vi "Big_LED_control.vi"() -> ()   [LabVIEW 2018]
uses:
  <instrlib>/niDCPower/nidcpower.llb/niDCPower Source Mode.ctl
  <instrlib>/niDCPower/nidcpower.llb/niDCPower Output Function.ctl
  AT lib/AmateurStepperMotor.dll
  <instrlib>/niDMM/nidmm.llb/niDMM Function.ctl
  <instrlib>/niDMM/nidmm.llb/niDMM Resolution in Digits.ctl
  <vilib>/Instr/_visa.llb/VISA Configure Serial Port (Instr).vi
  <instrlib>/niDMM/nidmm.llb/niDMM Configure Measurement Digits.vi
panel:
  in  "I - IV":bool
  in  "IV (gh)":bool
  in  "III (jk)":bool
  in  "II (Lm)":bool
  in  "I (np)":bool
  in  "Tab Control 2":enum32{"Шаговик и офир", "Служебная область"}(tab)
  in  "milliseconds to wait":u32=1000
  in  "Go To":dbl
  out "Ophir 1 Char":dbl(graph)=0.01
  in  "DecelerationTime, s":dbl=0.3
  in  "AccelerationTime, s":dbl=0.3
  in  "HoldOn":bool
  in  "Ophir 1 units":string(combo)="1000" caption="Units"
  out "Ophir 1 Over Range":bool caption="Over Range"
  out "Ophir 1 Optical Power":dbl=0.01 caption="Power" format="%#_4g"
  out "Ophir 1 MAX":dbl=0.01 caption="MAX" format="%#_5g"
  in  "Ophir 1 Clear":bool caption="Clear"
  in  "StepMultiplicationFactor":dbl=50.0
  in  "StepDivisor":i32(ring)=8 items=["D1"=1, "D2"=2, "D4"=4, "D8"=8, "D16"=16, "D32"=32]
  in  "Speed":dbl=250.0
  in  "Погнали!":bool
  in  "Стоп GoTo":bool
  out "Готово":bool
  out "Position":dbl=9.995
  in  "Ophir 1 Info":u16(ring)=1 caption="Info" items=["Device : JUNO; s/n:903793", "Head : PD300R-3W   ; s/n:779628"]
  in  "new pos":dbl
  in  "set pos":bool
  out "Device Response":string="*\n"
  in  "Ophir 1 usb channel":i16 caption="usb channel"
  out "Ophir 1 dup Visa Session":refnum<visa-resource-name>="USB0::0x0BD3::0x0777::NI-VISA-60003::RAW" caption="dup Visa Session"
  in  "Ophir 1 Baud Rate (3:9600)":i16(ring)=3 caption="Baud Rate (3:9600)" items=["300", "1200", "4800", "9600", "19200", "38400"]
  out "Ophir 1 Real Optical Power":dbl=1e-05 format="%.6e"
  in  "Ophir 1 GPIB Address (10)":string="10" caption="GPIB Address (10)"
  in  "Ophir 1 Port Number (default 2)":i16=1 caption="Port Number (default 2)" min=0 max=20
  in  "Ophir 1 Select Communication Protocol":u16(ring) caption="Select Communication Protocol" items=["USB", "RS232", "GPIB"]
  out "Ophir 1 error out":errorcluster caption="error out"
  in  "Ophir 1 error in (no error)":errorcluster caption="error in (no error)"
  in  "Ophir 1 Wait":u32=100 caption="Wait"
  out "IsOpen":bool=TRUE
  out "Ophir 1 Initialization":bool=TRUE caption="Initialization"
  in  "Tab Control":T1(tab)
  in  "POWER":bool
  in  "Стоп":bool
  in  "Resource Name":refnum<k15>="PXI1Slot2" caption="Источник питания"
  in  "Амперметр":refnum<k15>="PXI1Slot4" caption="NI DMM 1"
  in  "V_MB, V":dbl=6.0 caption="voltage level" min=0.0 max=6.0 format="%_6p"
  in  "curlim_V_MB, A":dbl=0.3 caption="current limit" format="%_6p"
  out "chart_0":dbl(graph)=-0.00013853853853977013 caption="Waveform Chart 5"
  in  "voltlim_I_LED, V":dbl=2.1 caption="current limit" min=0.01 format="%_6p"
  in  "I_LED, A":dbl=0.010000000000000004 caption="voltage level" format="%_6p"
  out "chart_1":dbl(graph)=-0.0002744397184121777 caption="Waveform Chart 5"
  out "Current Char":dbl(graph)=0.0055655837059021
  in  "Arduino":refnum<visa-resource-name>="COM16"
  in  "Сегменты":bool[](array[boolean])=[FALSE, FALSE, FALSE, FALSE, FALSE, FALSE, FALSE, FALSE, FALSE, FALSE, FALSE, FALSE, FALSE, FALSE, FALSE, FALSE, FALSE, FALSE]
  in  "Вольтметр":refnum<k15>="PXI1Slot5" caption="NI DMM 1"
  out "Voltage Char":dbl(graph)=0.2558511793613434
  in  "Port Name":string="COM8" caption="Порт шаговика"
  in  "wave_lenght":string="600"
  in  "Промер":bool caption="Промер сегмента"
  in  "NI DMM 1 Voltage Range 4":string(combo)="-1" caption="Range"
  in  "NI DMM 1 units 4":string(combo)="1" caption="Units"
  out "Voltage":dbl=0.2558511793613434 format="%_6g"
  in  "NI DMM 1 Current Range 3":string(combo)="1" caption="Range"
  in  "NI DMM 1 units 3":string(combo)="1000" caption="Units"
  out "Current":dbl=0.0055655837059021 format="%_6g"
  out "voltmes_V_MB, V":dbl=-0.00013853853853977013 caption="measurement" format="%_6g"
  out "curmes_V_MB, A":dbl=-0.0019423252169001965 caption="measurement" format="%_6g"
  out "curmes_I_LED, A":dbl=9.117163901385412e-07 caption="measurement" format="%_6g"
  out "voltmes_I_LED, V":dbl=-0.0002744397184121777 caption="measurement" format="%_6g"
  out "Разряд":dbl
  out "+/-":bool
  out "Power off":bool
  in  "Command":string="Cathode"
  in  "Записать":bool
  out "measure output \nfile refnum":refnum<file>
  out "Voltage, V":dbl=0.2558511793613434 caption="Measurement" format="%.5f"
  out "Current, A":dbl=5.5655837059021e-06 caption="Measurement" format="%.5f"
  out "Тип индикатора":string="Cathode"
  out "chart_2":dbl(graph)=0.0007584113885058215
  in  "V_RES, V":dbl caption="voltage level" format="%_6p"
  out "curmes_V_RES, A":dbl=9.838948216702391e-07 caption="measurement" format="%_6g"
  in  "curlim_V_RES, A":dbl=0.1 caption="current limit" min=0.01 format="%_6p"
  in  "measure path":path=path "C:/Users/user/Desktop/МСП/LabVIEW/LED_CONTROL_big_LED_ophir_24.12.24_1/Logs"
  out "Enum":enum16{"Exit", "4", "Промер", "2", "1"}(ring)
  out "№ об-ца":dbl
  out "Темп-ра":dbl
  out "Сегмент":string="n"
  out "voltmes_V_RES, V":dbl=0.0007584113885058215 caption="measurement" format="%_6g"
  in  "current level range":dbl=0.001 format="%#.6p"
  in  "1 - до 10 мА\n0 - от  30 мА":bool
  # "24.067"
  # "Шаговик"
  # "Офир"
  # "Шаговик"
  # "Офир"
  # "position - это значение абсолютное"
  # "j"
  # "c"
  # "d"
  # "e"
  # "g"
  # "h"
  # "a"
  # "b"
  # "f"
  # "k"
  # "L"
  # "m"
  # "n"
  # "p"
  # "dp"
  # "all"
  # "V_MB 5 В\nогрничение 300 м\n\nV_LED 2,1 В\nограничение 200 м"
  # "единицы мА\nrange 1 А"
  # "1. каждый сегмент включаем по отдельности, резистором постраиваем ток до 10 мА\n2. напряжение V_LED при этом не меняется\n3. в такоом положении промеряем сегменты по отдельности\n4. для промера всего индикатора сразу подстраиваем напряжение при неизменном положении резисторов\n5. ток всех индикаторов = ток одного сегмента (10 мА) * число сегментов (15)\n6. добиваемся этого увеличением V_LED"
  # "единицы В\nrange AUTO"
  # "регклировка суммарного тока через индикатор"
  # "24.063\n\n     I          U\n20 мА  1.3 В\n20 мА  1.4 В\n 7 мА   1.15 В"
  # "24.064\n\n     I          U\n10 мА  2 В\n10 мА  2.15 В\n 7 мА   1.9 В"
  # "автоматизировать подбор напряжения по известному максимальному напряжению и току. ОС по току сегмента"
  # "Р1:  +25°C\nР2:  - 60°C\nР3:  +85°C"
  # "регулировать ток в зависимости от температуры.\nс ростом температуры растет ток.\nпид-регулятор??"
  # "0. ввести номер образца\n1. включить нужный сегмент\n2. ввести его в поле справа\n3. вести температуру в поле слева\n4. нажать кнопку \"промер сегмента\""
  # "\"опрашивать кнопки не чаще, чем раз в секунду. сейчас кликать можно чаще, они загорятся, но ничего не произойдет\""
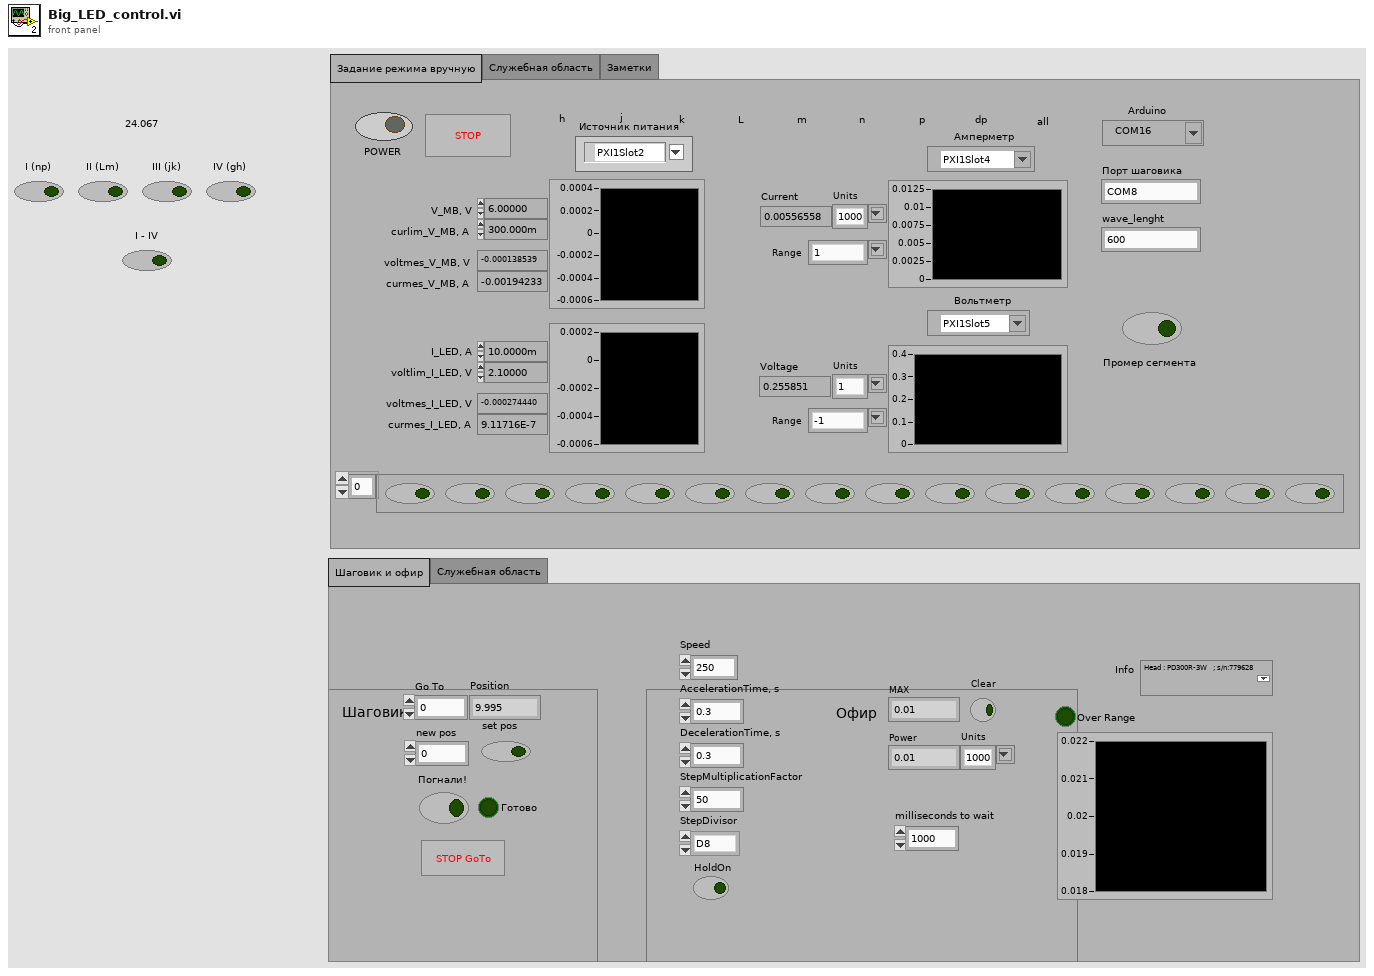
[diagram p1: front panel]
types:
  T1 = enum32{"Задание режима вручную", "Служебная область", "Заметки"}
  T2 = enum16{"open", "replace", "create", "open or create", "replace or create", "replace or create with confirmation"}
  T3 = typedef "niDCPower Output Function.ctl" = i32
  T4 = typedef "niDCPower Source Mode.ctl" = i32
  T5 = typedef "niDMM Function.ctl" = enum16{"DC Volts", "AC Volts", "DC Current", "AC Current", "2-wire Resistance", "4-wire Resistance", "Diode", "Frequency", "Period", "AC Volts DC Coupled", "Capacitance", "Inductance", "Temperature"}
  T6 = typedef "niDMM Resolution in Digits.ctl" = dbl
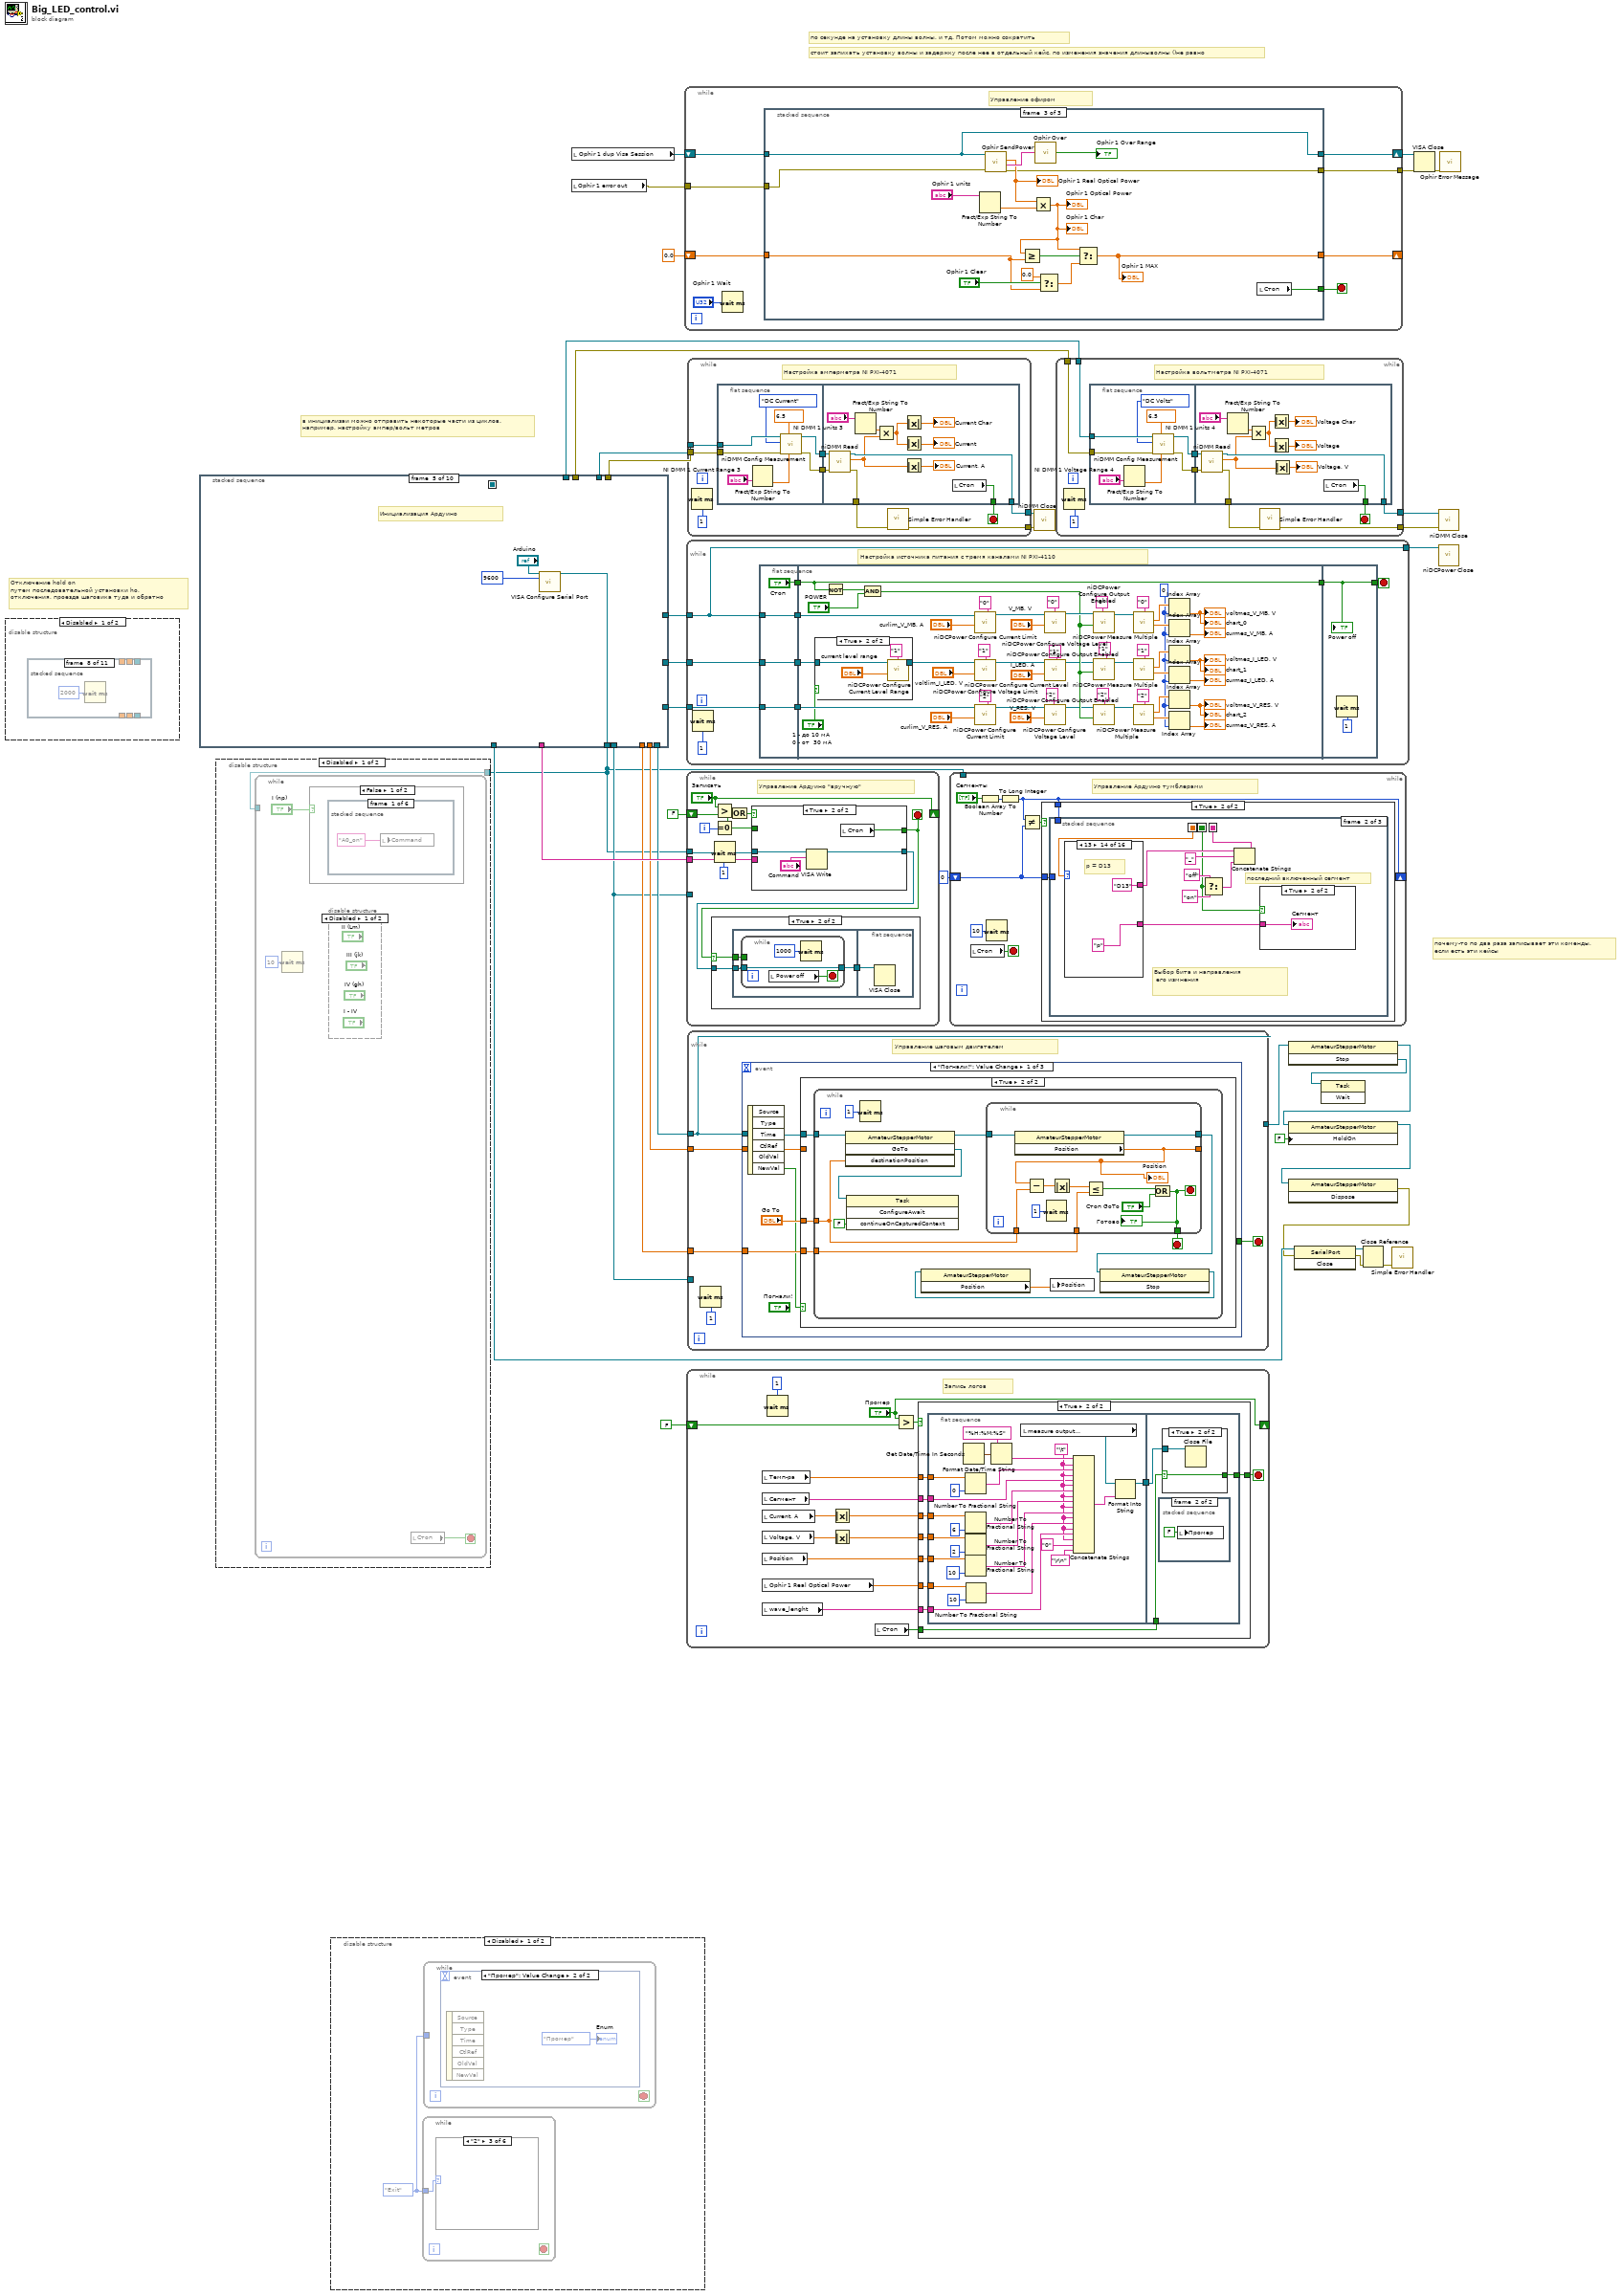
[diagram p0: block diagram]
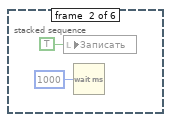
[diagram p3: hidden frame]
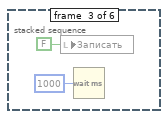
[diagram p4: hidden frame]
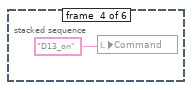
[diagram p5: hidden frame]
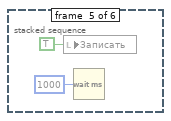
[diagram p6: hidden frame]
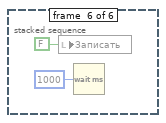
[diagram p7: hidden frame]
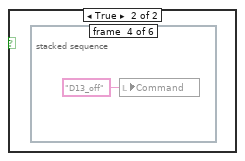
[diagram p8: hidden frame]
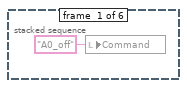
[diagram p9: hidden frame]
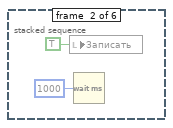
[diagram p10: hidden frame]
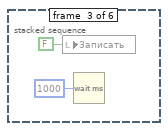
[diagram p11: hidden frame]
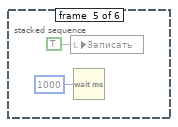
[diagram p12: hidden frame]
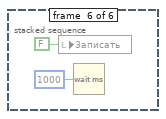
[diagram p13: hidden frame]
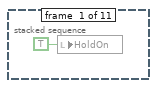
[diagram p15: hidden frame]
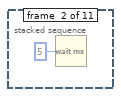
[diagram p16: hidden frame]
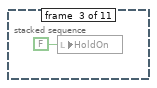
[diagram p17: hidden frame]
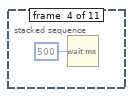
[diagram p18: hidden frame]
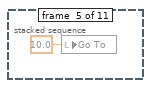
[diagram p19: hidden frame]
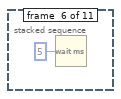
[diagram p20: hidden frame]
diagram:
  # "почему-то по два раза записывает эти коменды,\nесли есть эти кейсы"
  # "Отключение hold on\nпутем последовательной установки ho, \nотключения, проезда шаговика туда и обратно"
  # "в инициализаи можно отправить некоторые части из циклов.\nнапример, настройку ампер/вольт метров"
  # "стоит запихать установку волны и задержку после нее в отдельный кейс, по изменения значения длиныволны ()не равно"
  # "по секунде на установку длины волны, и тд. Потом можно сократить"
  n1 = disable-structure shown="Disabled" {
    frame Disabled {
      n2 = stacked-sequence {
        tunnel: _ -> [_ _ _ _ _ _ _ _ _ _ w50]
        tunnel: [_ _ _ _ _ _ _ _ _ _ w50] -> _
        tunnel: _ -> [_ _ _ _ _ _ _ _ _ _ w49]
        tunnel: [_ _ _ _ _ _ _ _ _ _ w49] -> _
        tunnel: [_ _ _ _ _ _ _ _ _ _ w48] -> _
        tunnel: _ -> [_ _ _ _ _ _ _ _ _ _ w48]
        frame #0 {
          n3 = local write "HoldOn"(TRUE ("HoldOn")) -> ()
        }
        frame #1 {
          n4 = Wait (ms)(milliseconds to wait=u32 5) -> ()  [unwired: 1 out]
        }
        frame #2 {
          n5 = local write "HoldOn"(FALSE ("HoldOn")) -> ()
        }
        frame #3 {
          n6 = Wait (ms)(milliseconds to wait=u32 500) -> ()  [unwired: 1 out]
        }
        frame #4 {
          n7 = local write "Go To"(10.0 ("Go To")) -> ()
        }
        frame #5 {
          n8 = Wait (ms)(milliseconds to wait=u32 5) -> ()  [unwired: 1 out]
        }
        frame #6 {
          n9 = local write "Погнали!"(TRUE ("Погнали!")) -> ()
        }
        frame #7 {
          n10 = Wait (ms)(milliseconds to wait=u32 2000) -> ()  [unwired: 1 out]
        }
        frame #8 {
          n11 = local write "Go To"(0.0 ("Go To")) -> ()
        }
        frame #9 {
          n12 = Wait (ms)(milliseconds to wait=u32 5) -> ()  [unwired: 1 out]
        }
        frame #10 {
          n13 = local write "Погнали!"(TRUE ("Погнали!")) -> ()
        }
      }
    }
    frame Enabled {
    }
  }
  n14 = stacked-sequence {
    seq-local: [_ _ _ _ _ _ w121 _ _ _] -> [_ _ _ _ _ _ _ w130 _ _]
    tunnel: [_ _ _ w68 _ _ _ _ _ _] -> w26
    tunnel: [_ w62 _ _ _ _ _ _ _ _] -> w37
    tunnel: [_ w61 _ _ _ _ _ _ _ _] -> w36
    tunnel: [_ _ _ _ w88 _ _ _ _ _] -> w1
    tunnel: [_ _ _ _ _ _ _ _ w136 _] -> w33
    tunnel: [_ _ w65 _ _ _ _ _ _ _] -> w32
    tunnel: [_ _ w64 _ _ _ _ _ _ _] -> w31
    tunnel: [_ _ _ _ _ _ _ w133 _ _] -> w3
    tunnel: [_ _ _ _ _ _ _ w131 _ _] -> w4
    tunnel: [_ _ _ _ _ _ _ w132 _ _] -> w5
    tunnel: [_ _ _ _ _ _ w111 _ _ _] -> w20
    tunnel: [_ _ _ w67 _ _ _ _ _ _] -> w8
    tunnel: [_ _ _ w66 _ _ _ _ _ _] -> w6
    tunnel: [_ _ _ _ _ _ _ _ _ w137] -> w2
    frame #0 {
      w52 = 0.0 ("currentmes_2")
      w53 = FALSE ("Стоп")
      # "ch 1"
      # "Обнуление переменных"
      n15 = local write "POWER"(w53) -> ()
      n16 = local write "Стоп"(w53) -> ()
      n17 = local write "+/-"(w53) -> ()
      n18 = local write "Погнали!"(w53) -> ()
      n19 = local write "Готово"(w53) -> ()
      n20 = local write "Стоп GoTo"(w53) -> ()
      n21 = local write "Промер"(w53) -> ()
      n22 = local write "curmes_V_MB, A"(w52) -> ()
      n23 = local write "voltmes_I_LED, V"(w52) -> ()
      n24 = local write "curmes_V_RES, A"(w52) -> ()
      n25 = local write "Current"(w52) -> ()
      n26 = local write "Разряд"(w52) -> ()
      n27 = local write "Go To"(w52) -> ()
      n28 = local write "Темп-ра"(w52) -> ()
      n29 = local write "№ об-ца"(w52) -> ()
      n30 = local write "Speed"(250.0 ("Speed")) -> ()
      n31 = local write "StepMultiplicationFactor"(50.0 ("StepMultiplicationFactor")) -> ()
      n32 = local write "AccelerationTime, s"(0.3 ("AccelerationTime, s")) -> ()
      n33 = local write "DecelerationTime, s"(0.3 ("DecelerationTime, s")) -> ()
      n34 = local write "current level range"(0.001 ("current level range")) -> ()
      n35 = local write "Сегменты"(bool[] [FALSE, FALSE, FALSE, FALSE, FALSE, FALSE, FALSE, FALSE, FALSE, FALSE, FALSE, FALSE, FALSE, FALSE, FALSE, FALSE, FALSE, FALSE] ("Сегменты")) -> ()
    }
    frame #1 {
      # "Инициализация амперметра"
      n36 = call <instrlib>:"niDMM Initialize.vi"("Instrument Descriptor"="Амперметр") -> ("error out"=w62:errorcluster, "instrument handle out"=w61:refnum<k15>)  [unwired: 9 in]
    }
    frame #2 {
      # "Инициализация вольтметра"
      n37 = call <instrlib>:"niDMM Initialize.vi"("Instrument Descriptor"="Вольтметр") -> ("error out"=w64:errorcluster, "instrument handle out"=w65:refnum<k15>)  [unwired: 9 in]
    }
    frame #3 {
      w73 = T3 1006 items=["DC Voltage"=1006, "DC Current"=1007, "Pulse Voltage"=1049, "Pulse Current"=1050] ("output function")
      w77 = T3 1007 items=["DC Voltage"=1006, "DC Current"=1007, "Pulse Voltage"=1049, "Pulse Current"=1050] ("output function")
      w78 = T3 1006 items=["DC Voltage"=1006, "DC Current"=1007, "Pulse Voltage"=1049, "Pulse Current"=1050] ("output function")
      w81 = T4 1020 items=["Single Point"=1020, "Sequence"=1021] ("source mode")
      # "Инициализация источника питания"
      n38 = call <instrlib>:"niDCPower Initialize.vi"("resource name"="Resource Name") -> ("instrument handle out"=w82:refnum<k15>)  [unwired: 3 in, 7 out]
      n39 = call <instrlib>:"niDCPower Configure Source Mode.vi"("source mode"=w81, "instrument handle"=w82) -> ("instrument handle out"=w72:refnum<k15>)  [unwired: 1 in, 8 out]
      n40 = call <instrlib>:"niDCPower Configure Output Function.vi"("output function"=w77, "channel name"="1", "instrument handle"=w72) -> ("instrument handle out"=w79:refnum<k15>)  [unwired: 7 in, 1 out]
      n41 = call <instrlib>:"niDCPower Configure Output Function.vi"("output function"=w73, "channel name"="2", "instrument handle"=w72) -> ("instrument handle out"=w74:refnum<k15>)  [unwired: 7 in, 1 out]
      n42 = call <instrlib>:"niDCPower Configure Output Function.vi"("output function"=w78, "channel name"="0", "instrument handle"=w72) -> ("instrument handle out"=w80:refnum<k15>)  [unwired: 7 in, 1 out]
      n43 = call <instrlib>:"niDCPower Configure Voltage Level.vi"("voltage level"=0.0, "channel name"="2", "instrument handle"=w74) -> ("instrument handle out"=w66:refnum<k15>)  [unwired: 7 in, 1 out]
      n44 = call <instrlib>:"niDCPower Configure Voltage Level.vi"("voltage level"=0.0, "channel name"="0", "instrument handle"=w80) -> ("instrument handle out"=w68:refnum<k15>)  [unwired: 7 in, 1 out]
      n45 = call <instrlib>:"niDCPower Configure Current Level.vi"("current level"=0.01, "channel name"="1", "instrument handle"=w79) -> ("instrument handle out"=w67:refnum<k15>)  [unwired: 7 in, 1 out]
    }
    frame #4 {
      # "Инициализация Ардуино"
      n46 = call-poly "VISA Configure Serial Port"("VISA resource name"="Arduino", "baud rate (9600)"=u32 9600) -> ("VISA resource name out"=w88:refnum<visa-resource-name>)  [unwired: 12 in, 1 out]
    }
    frame #5 {
      # "Инициализация офира"
      n47 = call "Ophir InitCom.vi"("GPIB Address (default 10)"="Ophir 1 GPIB Address (10)", "Communication (default USB 0)"="Ophir 1 Select Communication Protocol", "USB Channel number (default 0)"="Ophir 1 usb channel", "Port Number (default 2)"="Ophir 1 Port Number (default 2)", "error in (no error)"="Ophir 1 error in (no error)", "Baud Rate (3:9600)"="Ophir 1 Baud Rate (3:9600)") -> ("dup Visa Session"=w97:refnum<visa-resource-name>, "error out"=w96:errorcluster)  [unwired: 1 out]
      n48 = call "Ophir InstrInfo.vi"("Visa Session"=w97, "error in (no error)"=w96) -> ("dup Visa Session"=w109:refnum<visa-resource-name>, "Instrument Info"=w91:string, "error out"=w107:errorcluster)
      n49 = call "Ophir HeadInfo.vi"("Visa Session"=w109, "error in (no error)"=w107) -> ("error out"=w106:errorcluster, "dup Visa Session"=w108:refnum<visa-resource-name>, "Head Info"=w105:string)  [unwired: 6 out]
      n50 = call "Ophir InfoStrings.vi"("error in (no error)"=w106, "Head Info"=w105, "Instrument Info"=w91) -> ("error out"=w104:errorcluster, "Strings Array"=w103:string[])
      n51 = property on="Ophir 1 Info" class="Ring (strict)"("Strings []"=w103) -> ()  [unwired: 2 in, 2 out]
      n52 = call "Ophir ConfigDevice.vi"("Visa Session"=w108, "Measure Choice (0:Power)"=u16 0, "error in (no error)"=w104) -> ("dup Visa Session"=→"Ophir 1 dup Visa Session":refnum<visa-resource-name>, "OK ?"=→"Ophir 1 Initialization":bool, "error out"=→"Ophir 1 error out":errorcluster)  [unwired: 1 out]
    }
    frame #6 {
      w115 = 100 ("WriteTimeout")
      w120 = 1 items=["None", "One", "Two", "OnePointFive"] ("stopBits")
      w117 = 0 items=["None", "Odd", "Even", "Mark", "Space"] ("parity")
      # "убрали открытие порта. шаговик его и так сам откроет"
      # "Инициализация шаговика ч.1"
      n53 = constructor class="SerialPort"("portName"="Port Name", "baudRate"=57600, "parity"=w117, "dataBits"=8, "stopBits"=w120) -> (reference out=w114:refnum<k24>, error out=w113:errorcluster)  [unwired: 3 in, 6 out]
      n54 = property class="SerialPort"(reference=w114, error in=w113, "WriteTimeout"=w115, "ReadTimeout"=w115) -> (reference out=w111:refnum<k24>)  [unwired: 1 out]
      n55 = constructor class="AmateurStepperMotor"("serialPort"=w111) -> (reference out=w121:refnum<k24>, error out=w112:errorcluster)  [unwired: 3 in, 2 out]
      n56 = flat-sequence {
        tunnel: w112 -> [_]
        tunnel: w111 -> [w123]
        frame #0 {
          n57 = property class="SerialPort"(reference=w123) -> ("IsOpen"=→"IsOpen":bool)  [unwired: 1 in, 2 out]
        }
      }
    }
    frame #7 {
      # "стоит допустить изменение\nтих параметров в цикле, а не только \nпри инициализации"
      # "это те самые 50 шагов за мм"
      # "Инициализация шаговика ч.2"
      n58 = property class="AmateurStepperMotor"(reference=w130, "Speed"="Speed", "StepDivisor"="StepDivisor", "StepMultiplicationFactor"="StepMultiplicationFactor", "AccelerationTime"="AccelerationTime, s", "DecelerationTime"="DecelerationTime, s", "HoldOn"="HoldOn") -> (reference out=w133:refnum<k24>, "Position"=w131:dbl, "PositioningPrecision"=w132:dbl)  [unwired: 1 in, 1 out]
    }
    frame #8 {
      # "Begin VI: ОК или ОА?"
      n59 = call "Begin.vi"() -> ("Темп-ра"=→"Темп-ра":dbl, "№ об-ца"=→"№ об-ца":dbl, "String"=w136:string)  [unwired: 6 in]
      "Тип индикатора" <- w136
      n60 = local write "Command"(w136) -> ()
    }
    frame #9 {
      w147 = "\t"
      # "Инициализация логов"
      n61 = local read "№ об-ца"() -> (w151:dbl)
      n62 = Number To Fractional String(number=w151, precision (6)=i16 0) -> (F-format string=w152:string)  [unwired: 2 in]
      n63 = Get Date/Time In Seconds() -> (seconds since 1Jan1904=w162:timestamp)
      n64 = Build Path(base path="measure path", name or relative path=w152) -> (appended path=w158:path)
      n65 = call <vilib>:"Check if File or Folder Exists.vi"("path"=w158) -> ("file or folder exists?"=w159:bool, "dup path"=w160:path)  [unwired: 8 in, 1 out]
      n66 = Format Date/Time String(time format string (%c)="MES %d. %m. %y %H.%M.%S", seconds (now)=w162) -> (date/time string=w163:string)  [unwired: 1 in]
      n67 = case shown="True" w159 {
        tunnel: w160 -> [w169 w170]
        tunnel: [w168 w170] -> w161
        frame False {
          n68 = Create Folder(path (use dialog)=w169) -> (created path=w168:path)  [unwired: 2 in, 2 out]
        }
        frame True {
        }
      }
      n69 = Concatenate Strings(w163, ".xls" ("string")) -> (w164:string)
      n70 = Build Path(base path=w161, name or relative path=w164) -> (appended path=w165:path)
      n71 = Open/Create/Replace File(file path (use dialog)=w165, operation (0:open)=T2."open or create", access (0:read/write)=enum16{"read/write", "read-only", "write-only"}."read/write") -> (refnum out=w166:refnum<file>)  [unwired: 3 in, 2 out]
      n72 = Set File Position(refnum=w166, from (0:start)=enum16{"start", "end", "current"}."end") -> (refnum out=w149:refnum<file>)  [unwired: 2 in, 1 out]
      n73 = Format Into String(initial string=w149, "Time" ("string"), w147, "Temperature, C" ("string"), w147, "Segment" ("string"), w147, "Current, mA" ("string"), w147, "Voltage, V" ("input 7"), w147, "Distance, m" ("string"), w147, "Power, W " ("string"), w147, "Wavelenght, nm" ("input 17"), w147, "Candlepower, kd" ("string"), "\r\n") -> (resulting string=w137:refnum<file>)  [unwired: 2 in, 1 out]
      "measure output \nfile refnum" <- w137
    }
  }
  n74 = disable-structure shown="Disabled" {
    disable-tunnel: w1 -> [w171 _]
    frame Disabled {
      n75 = while {
        tunnel: w171 -> [_]
        stop <- w173 stop-if-true
        n76 = Wait (ms)(milliseconds to wait=u32 10 ("millisecond timer value")) -> ()  [unwired: 1 out]
        n77 = case shown="False" "I (np)" {
          frame False {
            n78 = stacked-sequence {
              frame #0 {
                n79 = local write "Command"("A0_on" ("Command")) -> ()
              }
              frame #1 {
                n80 = local write "Записать"(TRUE ("Записать")) -> ()
                n81 = Wait (ms)(milliseconds to wait=u32 1000) -> ()  [unwired: 1 out]
              }
              frame #2 {
                n82 = local write "Записать"(FALSE ("Записать")) -> ()
                n83 = Wait (ms)(milliseconds to wait=u32 1000) -> ()  [unwired: 1 out]
              }
              frame #3 {
                n84 = local write "Command"("D13_on" ("Command")) -> ()
              }
              frame #4 {
                n85 = local write "Записать"(TRUE ("Записать")) -> ()
                n86 = Wait (ms)(milliseconds to wait=u32 1000) -> ()  [unwired: 1 out]
              }
              frame #5 {
                n87 = local write "Записать"(FALSE ("Записать")) -> ()
                n88 = Wait (ms)(milliseconds to wait=u32 1000) -> ()  [unwired: 1 out]
              }
            }
          }
          frame True {
            n89 = stacked-sequence {
              frame #0 {
                n90 = local write "Command"("A0_off" ("Command")) -> ()
              }
              frame #1 {
                n91 = local write "Записать"(TRUE ("Записать")) -> ()
                n92 = Wait (ms)(milliseconds to wait=u32 1000) -> ()  [unwired: 1 out]
              }
              frame #2 {
                n93 = local write "Записать"(FALSE ("Записать")) -> ()
                n94 = Wait (ms)(milliseconds to wait=u32 1000) -> ()  [unwired: 1 out]
              }
              frame #3 {
                n95 = local write "Command"("D13_off" ("Command")) -> ()
              }
              frame #4 {
                n96 = local write "Записать"(TRUE ("Записать")) -> ()
                n97 = Wait (ms)(milliseconds to wait=u32 1000) -> ()  [unwired: 1 out]
              }
              frame #5 {
                n98 = local write "Записать"(FALSE ("Записать")) -> ()
                n99 = Wait (ms)(milliseconds to wait=u32 1000) -> ()  [unwired: 1 out]
              }
            }
          }
        }
        n100 = disable-structure shown="Disabled" {
          frame Disabled {
          }
          frame Enabled {
          }
        }
        n101 = local read "Стоп"() -> (w173:bool)
      }
    }
    frame Enabled {
    }
  }
  n102 = disable-structure shown="Disabled" {
    frame Disabled {
      w195 = enum16{"Exit", "4", "Промер", "2", "1"}."Exit"
      n103 = while {
        tunnel: w195 -> [w196]
        stop <- _ stop-if-true
        n104 = case shown="\"2\"" w196 {
          frame "Exit", Default {
          }
          frame "4" {
          }
          frame "2" {
          }
          frame "2" {
          }
          frame "1" {
          }
          frame "Промер" {
          }
        }
      }
      n105 = while {
        tunnel: w195 -> [_]
        stop <- _ stop-if-true
        n106 = event shown="[1] \"Промер\": Value Change" {
          selector: _ -> [_ _]
          dyn-events: _ -> [_ _]
          timeout: _ -> [_ _]
          event Timeout {
            n107 = event-data() -> ()  [unwired: 1 in, 3 out]
          }
          event "Промер": Value Change {
            n108 = event-data() -> ()  [unwired: 1 in, 6 out]
            "Enum" <- enum16{"Exit", "4", "Промер", "2", "1"}."Промер" ("Enum")
          }
        }
      }
    }
    frame Enabled {
    }
  }
  n109 = local read "Ophir 1 error out"() -> (w24:errorcluster)
  n110 = local read "Ophir 1 dup Visa Session"() -> (w25:refnum<visa-resource-name>)
  n111 = while {
    tunnel: w24 -> [w204]
    shift-right: [w200] -> _
    shift-left: 0.0 ("t") -> [w203]
    shift-right: [w201] -> w18
    shift-left: w25 -> [w205]
    tunnel: [w199] -> w17
    stop <- w198 stop-if-true
    # "Управление офиром"
    n112 = Wait (ms)(milliseconds to wait="Ophir 1 Wait") -> ()  [unwired: 1 out]
    n113 = stacked-sequence {
      tunnel: w205 -> [w209 _ w212]
      tunnel: w204 -> [w208 _ w214]
      tunnel: w203 -> [_ _ w215]
      tunnel: [_ _ w212] -> w201
      tunnel: [_ _ w216] -> w200
      tunnel: [_ _ w213] -> w199
      tunnel: [_ _ w211] -> w198
      frame #0 {
        n114 = call "light_setWaveLenght.vi"("error in (no error)"=w208, "Visa Session"=w209, "wave_lenght"="wave_lenght") -> ("Device Response"=→"Device Response":string)  [unwired: 6 in, 2 out]
      }
      frame #1 {
        n115 = Wait (ms)(milliseconds to wait="milliseconds to wait") -> ()  [unwired: 1 out]
      }
      frame #2 {
        n116 = Fract/Exp String To Number(string="Ophir 1 units") -> (number=w219:dbl)  [unwired: 3 in, 1 out]
        n117 = call "Ophir SendPower.vi"("Visa Session"=w212, "error in (no error)"=w214) -> ("Value Number"=w218:dbl, "Value String"=w225:string, "error out"=w213:errorcluster)  [unwired: 1 out]
        "Ophir 1 Real Optical Power" <- w218
        n118 = Multiply(x=w218, y=w219) -> (x*y=w222:dbl)
        "Ophir 1 Char" <- w222
        "Ophir 1 Optical Power" <- w222
        n119 = Greater Or Equal?(x=w222, y=w215) -> (x >= y?=w223:bool)
        n120 = call "Ophir Over.vi"("Value String"=w225) -> ("Overrange"=→"Ophir 1 Over Range":bool)
        n121 = Select(t=0.0, s="Ophir 1 Clear", f=w215) -> (s? t:f=w221:dbl)
        n122 = Select(t=w222, s=w223, f=w221) -> (s? t:f=w216:dbl)
        "Ophir 1 MAX" <- w216
        n123 = local read "Стоп"() -> (w211:bool)
      }
    }
  }
  n124 = while {
    tunnel: w26 -> [w233]
    tunnel: [w233] -> w34
    tunnel: w8 -> [w230]
    tunnel: w6 -> [w227]
    stop <- w229 stop-if-true
    # "Настройка источника питания с тремя каналами NI PXI-4110"
    n125 = Wait (ms)(milliseconds to wait=u32 1) -> ()  [unwired: 1 out]
    n126 = flat-sequence {
      tunnel: w233 -> [w240]
      tunnel: [w240] -> w235
      tunnel: ["Стоп"] -> w234
      tunnel: [w238] -> w231
      tunnel: w230 -> [w238]
      tunnel: [w237] -> w228
      tunnel: w227 -> [w237]
      tunnel: w235 -> [w285]
      tunnel: w234 -> [w289]
      tunnel: [w289] -> w232
      tunnel: w231 -> [w253]
      tunnel: w228 -> [w248]
      tunnel: [w296] -> w229
      tunnel: w232 -> [w296]
      frame #0 {
      }
      frame #1 {
        w254 = 0 ("index")
        n127 = case shown="True" "1 - до 10 мА\n0 - от  30 мА" {
          tunnel: w253 -> [w290 w294]
          tunnel: [w290 w293] -> w252
          frame False {
          }
          frame True {
            n128 = call <instrlib>:"niDCPower Configure Current Level Range.vi"("current level range"="current level range", "channel name"="1", "instrument handle"=w294) -> ("instrument handle out"=w293:refnum<k15>)  [unwired: 7 in, 1 out]
          }
        }
        n129 = Not(x=w289) -> (.not. x?=w288:bool)
        n130 = And(x=w288, y="POWER") -> (x .and. y?=w284:bool)
        n131 = call <instrlib>:"niDCPower Configure Current Limit.vi"("current limit"="curlim_V_MB, A", "channel name"="0", "instrument handle"=w285) -> ("instrument handle out"=w275:refnum<k15>)  [unwired: 7 in, 1 out]
        n132 = call <instrlib>:"niDCPower Configure Voltage Limit.vi"("voltage limit"="voltlim_I_LED, V", "channel name"="1", "instrument handle"=w252) -> ("instrument handle out"=w279:refnum<k15>)  [unwired: 7 in, 1 out]
        n133 = call <instrlib>:"niDCPower Configure Current Limit.vi"("current limit"="curlim_V_RES, A", "channel name"="2", "instrument handle"=w248) -> ("instrument handle out"=w269:refnum<k15>)  [unwired: 7 in, 1 out]
        n134 = call <instrlib>:"niDCPower Configure Voltage Level.vi"("voltage level"="V_MB, V", "channel name"="0", "instrument handle"=w275) -> ("instrument handle out"=w286:refnum<k15>)  [unwired: 7 in, 1 out]
        n135 = call <instrlib>:"niDCPower Configure Current Level.vi"("current level"="I_LED, A", "channel name"="1", "instrument handle"=w279) -> ("instrument handle out"=w280:refnum<k15>)  [unwired: 7 in, 1 out]
        n136 = call <instrlib>:"niDCPower Configure Voltage Level.vi"("voltage level"="V_RES, V", "channel name"="2", "instrument handle"=w269) -> ("instrument handle out"=w270:refnum<k15>)  [unwired: 7 in, 1 out]
        n137 = call <instrlib>:"niDCPower Configure Output Enabled.vi"("output enabled"=w284, "channel name"="0", "instrument handle"=w286) -> ("instrument handle out"=w263:refnum<k15>)  [unwired: 7 in, 1 out]
        n138 = call <instrlib>:"niDCPower Configure Output Enabled.vi"("output enabled"=w284, "channel name"="1", "instrument handle"=w280) -> ("instrument handle out"=w256:refnum<k15>)  [unwired: 7 in, 1 out]
        n139 = call <instrlib>:"niDCPower Configure Output Enabled.vi"("output enabled"=w284, "channel name"="2", "instrument handle"=w270) -> ("instrument handle out"=w255:refnum<k15>)  [unwired: 7 in, 1 out]
        n140 = call <instrlib>:"niDCPower Measure Multiple.vi"("channel name"="0", "instrument handle"=w263) -> ("current measurements"=w261:dbl[], "voltage measurements"=w262:dbl[])  [unwired: 6 in, 2 out]
        n141 = call <instrlib>:"niDCPower Measure Multiple.vi"("channel name"="1", "instrument handle"=w256) -> ("current measurements"=w259:dbl[], "voltage measurements"=w260:dbl[])  [unwired: 6 in, 2 out]
        n142 = call <instrlib>:"niDCPower Measure Multiple.vi"("channel name"="2", "instrument handle"=w255) -> ("current measurements"=w257:dbl[], "voltage measurements"=w258:dbl[])  [unwired: 6 in, 2 out]
        n143 = Index Array(array=w262, index=w254) -> (element=→"chart_0" →"voltmes_V_MB, V":dbl)
        n144 = Index Array(array=w261, index=w254) -> (element=→"curmes_V_MB, A":dbl)
        n145 = Index Array(array=w260, index=w254) -> (element=→"chart_1" →"voltmes_I_LED, V":dbl)
        n146 = Index Array(array=w259, index=w254) -> (element=→"curmes_I_LED, A":dbl)
        n147 = Index Array(array=w258, index=w254) -> (element=→"chart_2" →"voltmes_V_RES, V":dbl)
        n148 = Index Array(array=w257, index=w254) -> (element=→"curmes_V_RES, A":dbl)
      }
      frame #2 {
        n149 = Wait (ms)(milliseconds to wait=u32 1) -> ()  [unwired: 1 out]
        "Power off" <- w296
      }
    }
  }
  n150 = while {
    tunnel: w1 -> [w304]
    shift-right: ["Записать"] -> _
    shift-left: FALSE ("Записать") -> [w306]
    tunnel: w33 -> [w302]
    tunnel: w2 -> [_]
    i -> [w303]
    stop <- w297 stop-if-true
    # "Управление Ардуино \"вручную\""
    n151 = Greater?(x="Записать", y=w306) -> (0:w300:bool)
    n152 = Equal To 0?(x=w303) -> (x = 0?=w299:bool)
    n153 = Wait (ms)(milliseconds to wait=u32 1) -> ()  [unwired: 1 out]
    n154 = Or(x=w300, y=w299) -> (x .or. y?=w301:bool)
    n155 = case shown="True" w301 {
      tunnel: w304 -> [w318 w323]
      tunnel: [w319 w322] -> w297
      tunnel: w302 -> [_ _]
      tunnel: w299 -> [_ _]
      tunnel: [w318 w320] -> w298
      frame False {
        n156 = local read "Стоп"() -> (w319:bool)
      }
      frame True {
        n157 = VISA Write(VISA resource name=w323, write buffer="Command") -> (VISA resource name out=w320:refnum<visa-resource-name>)  [unwired: 1 in, 2 out]
        n158 = local read "Стоп"() -> (w322:bool)
      }
    }
    n159 = case shown="True" w297 {
      selector: w297 -> [_ w308]
      tunnel: w298 -> [_ w310]
      frame False {
      }
      frame True {
        n160 = flat-sequence {
          tunnel: w310 -> [w313]
          tunnel: [w312] -> w309
          tunnel: w308 -> [w311]
          tunnel: w309 -> [w317]
          frame #0 {
            n161 = while {
              tunnel: w313 -> [w316]
              tunnel: [w316] -> w312
              tunnel: w311 -> [_]
              stop <- w314 stop-if-true
              n162 = local read "Power off"() -> (w314:bool)
              n163 = Wait (ms)(milliseconds to wait=u32 1000) -> ()  [unwired: 1 out]
            }
          }
          frame #1 {
            n164 = VISA Close(VISA resource name=w317) -> ()  [unwired: 1 in, 1 out]
          }
        }
      }
    }
  }
  n165 = while {
    shift-right: ["Промер"] -> _
    shift-left: FALSE ("Промер сегмента") -> [w336]
    stop <- w333 stop-if-true
    # "Запиcь логов"
    n166 = local read "Темп-ра"() -> (w329:dbl)
    n167 = local read "Сегмент"() -> (w330:string)
    n168 = local read "Current, A"() -> (w332:dbl)
    n169 = local read "Voltage, V"() -> (w331:dbl)
    n170 = local read "Position"() -> (w328:dbl)
    n171 = local read "Ophir 1 Real Optical Power"() -> (w326:dbl)
    n172 = local read "wave_lenght"() -> (w327:string)
    n173 = Wait (ms)(milliseconds to wait=u32 1) -> ()  [unwired: 1 out]
    n174 = Absolute Value(x=w332) -> (abs(x)=w324:dbl)
    n175 = Absolute Value(x=w331) -> (abs(x)=w325:dbl)
    n176 = local read "Стоп"() -> (w334:bool)
    n177 = Greater?(x="Промер", y=w336) -> (0:w337:bool)
    n178 = case shown="True" w337 {
      tunnel: w324 -> [_ w349]
      tunnel: w325 -> [_ w348]
      tunnel: w328 -> [_ w345]
      tunnel: w326 -> [_ w346]
      tunnel: w327 -> [_ w347]
      tunnel: w334 -> [w339 w343]
      tunnel: w329 -> [_ w342]
      tunnel: w330 -> [_ w341]
      tunnel: [w339 w340] -> w333
      frame False {
      }
      frame True {
        n179 = flat-sequence {
          tunnel: w349 -> [w367]
          tunnel: w348 -> [w366]
          tunnel: w347 -> [w364]
          tunnel: w346 -> [w363]
          tunnel: w345 -> [w362]
          tunnel: [w357] -> w344
          tunnel: w342 -> [w356]
          tunnel: w341 -> [w350]
          tunnel: w344 -> [w378]
          tunnel: w343 -> [w377]
          tunnel: [w376] -> w340
          frame #0 {
            w352 = "\t"
            n180 = Get Date/Time In Seconds() -> (seconds since 1Jan1904=w375:timestamp)
            n181 = Number To Fractional String(number=w356, precision (6)=i16 0) -> (F-format string=w354:string)  [unwired: 2 in]
            n182 = Number To Fractional String(number=w367, precision (6)=i16 6) -> (F-format string=w370:string)  [unwired: 2 in]
            n183 = Number To Fractional String(number=w366, precision (6)=i16 2) -> (F-format string=w369:string)  [unwired: 2 in]
            n184 = Number To Fractional String(number=w362, precision (6)=i16 10) -> (F-format string=w368:string)  [unwired: 2 in]
            n185 = Number To Fractional String(number=w363, precision (6)=i16 10) -> (F-format string=w365:string)  [unwired: 2 in]
            n186 = Format Date/Time String(time format string (%c)="%H:%M:%S", seconds (now)=w375) -> (date/time string=w373:string)  [unwired: 1 in]
            n187 = local read "measure output \nfile refnum"() -> (w371:refnum<file>)
            n188 = Concatenate Strings(w373, w352, w354, w352, w350, w352, w370, w352, w369, w352, w368, w352, w365, w352, w364, w352, "0" ("string"), "\r\n") -> (w372:string)
            n189 = Format Into String(initial string=w371, w372) -> (resulting string=w357:refnum<file>)  [unwired: 2 in, 1 out]
          }
          frame #1 {
            n190 = stacked-sequence {
              frame #0 {
                n191 = Wait (ms)(milliseconds to wait=u32 250) -> ()  [unwired: 1 out]
              }
              frame #1 {
                n192 = local write "Промер"(FALSE ("Промер")) -> ()
              }
            }
            n193 = case shown="True" w377 {
              selector: w377 -> [_ w382]
              tunnel: w378 -> [_ w383]
              tunnel: [FALSE w382] -> w376
              frame False {
              }
              frame True {
                n194 = Close File(refnum=w383) -> ()  [unwired: 1 in, 2 out]
              }
            }
          }
        }
      }
    }
  }
  n195 = while {
    tunnel: [w390] -> w27
    tunnel: w36 -> [w388]
    tunnel: w37 -> [w387]
    tunnel: [w384] -> w28
    stop <- w386 stop-if-true
    # "Настройка амперметра NI PXI-4071"
    n196 = Wait (ms)(milliseconds to wait=u32 1) -> ()  [unwired: 1 out]
    n197 = flat-sequence {
      tunnel: [w397] -> w392
      tunnel: w388 -> [w395]
      tunnel: w387 -> [w399]
      tunnel: [w396] -> w391
      tunnel: w392 -> [w409]
      tunnel: w391 -> [w412]
      tunnel: [w408] -> w386
      tunnel: [w407] -> w384
      tunnel: [w406] -> w385
      frame #0 {
        w393 = T6 6.5 items=["3 1/2"=3.5, "4 1/2"=4.5, "5 1/2"=5.5, "6 1/2"=6.5, "7 1/2"=7.5] ("Resolution in Digits")
        n198 = Fract/Exp String To Number(string="NI DMM 1 Current Range 3") -> (number=w398:dbl)  [unwired: 3 in, 1 out]
        n199 = call-poly <instrlib>:"niDMM Config Measurement.vi"("Range"=w398, "Resolution in Digits"=w393, "error in (no error)"=w399, "Function"=niDMM_Function."DC Current" ("Measurement Type"), "instrument handle"=w395) -> ("error out"=w396:errorcluster, "instrument handle out"=w397:refnum<k15>)  [unwired: 5 in]
      }
      frame #1 {
        n200 = call <instrlib>:"niDMM Read.vi"("error in (no error)"=w412, "instrument handle"=w409) -> ("error out"=w406:errorcluster, "Measurement"=w401:dbl, "instrument handle out"=w407:refnum<k15>)  [unwired: 7 in]
        n201 = Fract/Exp String To Number(string="NI DMM 1 units 3") -> (number=w410:dbl)  [unwired: 3 in, 1 out]
        n202 = Multiply(x=w410, y=w401) -> (x*y=w403:dbl)
        n203 = Absolute Value(x=w403) -> (abs(x)=→"Current Char":dbl)
        n204 = Absolute Value(x=w403) -> (abs(x)=→"Current":dbl)
        n205 = Absolute Value(x=w401) -> (abs(x)=→"Current, A":dbl)
        n206 = local read "Стоп"() -> (w408:bool)
      }
    }
    n207 = call <vilib>:"Simple Error Handler.vi"("error in (no error)"=w385) -> ("error out"=w390:errorcluster)  [unwired: 1 in, 7 out]
  }
  n208 = while {
    tunnel: w3 -> [w414]
    tunnel: w5 -> [w416]
    tunnel: [w414] -> w7
    tunnel: w4 -> [w417]
    tunnel: w2 -> [_]
    stop <- w413 stop-if-true
    # "Управление шаговым двигателем"
    n209 = Wait (ms)(milliseconds to wait=u32 1) -> ()  [unwired: 1 out]
    n210 = event shown="[0] \"Погнали!\": Value Change" {
      selector: _ -> [_ _ _]
      dyn-events: _ -> [_ _ _]
      timeout: _ -> [_ _ _]
      tunnel: w414 -> [w422 w450 _]
      tunnel: w417 -> [w421 _ _]
      tunnel: w416 -> [w420 _ _]
      tunnel: [_ _ w456] -> w413
      event "Погнали!": Value Change {
        n211 = event-data() -> ("NewVal"=w418:bool)  [unwired: 1 in, 5 out]
        n212 = case shown="True" w418 {
          tunnel: "Go To" -> [_ w426]
          tunnel: w422 -> [_ w425]
          tunnel: w421 -> [_ _]
          tunnel: w420 -> [_ w424]
          frame False {
            n213 = Wait (ms)(milliseconds to wait=u32 1) -> ()  [unwired: 1 out]
          }
          frame True {
            n214 = while {
              tunnel: w426 -> [w433]
              tunnel: w425 -> [w434]
              tunnel: w424 -> [w436]
              stop <- w437 stop-if-true
              n215 = invoke class="AmateurStepperMotor" method="GoTo"(reference=w434, "destinationPosition"=w433) -> (reference out=w429:refnum<k24>, "GoTo"=w432:refnum<k24>)  [unwired: 2 in, 2 out]
              n216 = invoke class="Task" method="ConfigureAwait"(reference=w432, "continueOnCapturedContext"=FALSE) -> ()  [unwired: 2 in, 4 out]
              n217 = Wait (ms)(milliseconds to wait=u32 1) -> ()  [unwired: 1 out]
              n218 = while {
                tunnel: [w438] -> _
                tunnel: [w440] -> w430
                tunnel: [w442] -> w437
                tunnel: w433 -> [w447]
                tunnel: w436 -> [w445]
                tunnel: w429 -> [w439]
                stop <- w442 stop-if-true
                n219 = property class="AmateurStepperMotor"(reference=w439) -> (reference out=w440:refnum<k24>, "Position"=w438:dbl)  [unwired: 1 in, 1 out]
                "Position" <- w438
                n220 = Subtract(x=w438, y=w447) -> (x-y=w448:dbl)
                n221 = Wait (ms)(milliseconds to wait=u32 1) -> ()  [unwired: 1 out]
                n222 = Absolute Value(x=w448) -> (abs(x)=w446:dbl)
                n223 = Less Or Equal?(x=w446, y=w445) -> (x <= y?=w444:bool)
                n224 = Or(x=w444, y="Стоп GoTo") -> (x .or. y?=w442:bool)
                "Готово" <- w442
              }
              n225 = invoke class="AmateurStepperMotor" method="Stop"(reference=w430) -> (reference out=w428:refnum<k24>)  [unwired: 2 in, 2 out]
              n226 = property class="AmateurStepperMotor"(reference=w428) -> ("Position"=w427:dbl)  [unwired: 1 in, 2 out]
              n227 = local write "Position"(w427) -> ()
            }
          }
        }
      }
      event "set pos": Value Change {
        n228 = event-data() -> ("NewVal"=w451:bool)  [unwired: 1 in, 5 out]
        n229 = case shown="False" w451 {
          tunnel: w450 -> [_ w455]
          tunnel: "new pos" -> [_ w454]
          frame False {
          }
          frame True {
            n230 = property class="AmateurStepperMotor"(reference=w455, "Position"=w454) -> (reference out=w453:refnum<k24>)  [unwired: 1 in, 1 out]
            n231 = property class="AmateurStepperMotor"(reference=w453) -> ("Position"=w452:dbl)  [unwired: 1 in, 2 out]
            n232 = local write "Position"(w452) -> ()
          }
        }
      }
      event "Стоп": Value Change {
        n233 = event-data() -> ()  [unwired: 1 in, 6 out]
        n234 = local read "Стоп"() -> (w456:bool)
      }
    }
  }
  n235 = while {
    shift-right: [w457] -> _
    shift-left: 0 -> [w459]
    tunnel: w1 -> [_]
    stop <- w463 stop-if-true
    # "Управление Ардуино тумблерами"
    n236 = local read "Стоп"() -> (w463:bool)
    n237 = Boolean Array To Number(Boolean array="Сегменты") -> (number=w458:u32)
    n238 = Wait (ms)(milliseconds to wait=u32 10 ("millisecond timer value")) -> ()  [unwired: 1 out]
    n239 = To Long Integer(number=w458) -> (32bit integer=w457:i32)
    n240 = Not Equal?(x=w457, y=w459) -> (x != y?=w461:bool)
    n241 = case shown="True" w461 {
      tunnel: w457 -> [_ w464]
      tunnel: w459 -> [_ w465]
      frame False {
      }
      frame True {
        n242 = stacked-sequence {
          seq-local: [w468 _ _] -> [_ w473 _]
          seq-local: [w466 _ _] -> [_ w477 _]
          seq-local: [_ w478 _] -> [_ _ w515]
          tunnel: w464 -> [w470 _ _]
          tunnel: w465 -> [w469 _ _]
          frame #0 {
            # "Детектирвоание позиции и\nнаправления изменения бита"
            n243 = Subtract(x=w470, y=w469) -> (x-y=w471:i32)
            n244 = To Double Precision Float(number=w471) -> (double precision float=w472:dbl)
            n245 = Greater Than 0?(x=w471) -> (x > 0?=w468:bool)
            "+/-" <- w468
            n246 = Absolute Value(x=w472) -> (abs(x)=w467:dbl)
            n247 = Logarithm Base 2(1:w467) -> (0:w466:dbl)
            "Разряд" <- w466
          }
          frame #1 {
            # "последний включенный сегмент"
            # "Выбор бита и направления\n его измнения"
            n248 = case shown="13" w477 {
              tunnel: ["D10" "D9" "D5" "D8" "D11" "D12" "A1" "D4" "A5" "A4" "A3" "A2" "A0" "D13" "D3" "All"] -> w475
              tunnel: ["a" "b" "c" "d" "e" "f" "g" "h" "j" "k" "L" "m" "n" "p" "dp" "All"] -> w474
              frame 0, Default {
                # "a = D10"
              }
              frame 1 {
                # "b = D9"
              }
              frame 2 {
                # "c = D5"
              }
              frame 3 {
                # "d = D8"
              }
              frame 4 {
                # "e = D11"
              }
              frame 5 {
                # "f = D12"
              }
              frame 6 {
                # "g = A1"
              }
              frame 7 {
                # "h = D4"
              }
              frame 8 {
                # "j = A5"
              }
              frame 9 {
                # "k = A4"
              }
              frame 10 {
                # "L = A3"
              }
              frame 11 {
                # "m = A2"
              }
              frame 12 {
                # "n = A0"
              }
              frame 13 {
                # "p = D13"
              }
              frame 14 {
                # "dp = D3"
              }
              frame 15 {
              }
            }
            n249 = Select(t="off", s=w473, f="on") -> (s? t:f=w476:string)
            n250 = Concatenate Strings(w475, "_" ("string"), w476) -> (w478:string)
            n251 = case shown="True" w473 {
              tunnel: w474 -> [_ w482]
              frame False {
              }
              frame True {
                "Сегмент" <- w482
              }
            }
          }
          frame #2 {
            # "Передача команды в Ардуино"
            n252 = disable-structure shown="Disabled" {
              disable-tunnel: w515 -> [w517 _]
              frame Disabled {
                n253 = Equal?(x=w517, y="All_off") -> (x = y?=w520:bool)
                n254 = Equal?(x=w517, y="All_on") -> (x = y?=w518:bool)
                n255 = case shown="True" w520 {
                  frame False {
                  }
                  frame True {
                    n256 = local write "Сегменты"(bool[] [TRUE, TRUE, TRUE, TRUE, TRUE, TRUE, TRUE, TRUE, TRUE, TRUE, TRUE, TRUE, TRUE, TRUE, TRUE, TRUE] ("Сегменты")) -> ()
                  }
                }
                n257 = case shown="True" w518 {
                  frame False {
                  }
                  frame True {
                    n258 = local write "Сегменты"(bool[] [FALSE, FALSE, FALSE, FALSE, FALSE, FALSE, FALSE, FALSE, FALSE, FALSE, FALSE, FALSE, FALSE, FALSE, FALSE, FALSE] ("Сегменты")) -> ()
                  }
                }
              }
              frame Enabled {
              }
            }
            n259 = stacked-sequence {
              tunnel: w515 -> [w523 _ _]
              frame #0 {
                n260 = local write "Command"(w523) -> ()
              }
              frame #1 {
                n261 = local write "Записать"(TRUE ("Записать")) -> ()
                n262 = Wait (ms)(milliseconds to wait=u32 1000) -> ()  [unwired: 1 out]
              }
              frame #2 {
                n263 = local write "Записать"(FALSE ("Записать")) -> ()
                n264 = Wait (ms)(milliseconds to wait=u32 1000) -> ()  [unwired: 1 out]
              }
            }
          }
        }
      }
    }
  }
  n265 = call <instrlib>:"niDMM Close.vi"("error in (no error)"=w27, "instrument handle"=w28) -> ()  [unwired: 9 in, 1 out]
  n266 = while {
    tunnel: [w534] -> w29
    tunnel: w32 -> [w532]
    tunnel: w31 -> [w531]
    tunnel: [w528] -> w30
    stop <- w530 stop-if-true
    # "Настройка вольтметра NI PXI-4071"
    n267 = Wait (ms)(milliseconds to wait=u32 1) -> ()  [unwired: 1 out]
    n268 = flat-sequence {
      tunnel: [w541] -> w536
      tunnel: w532 -> [w539]
      tunnel: w531 -> [w543]
      tunnel: [w540] -> w535
      tunnel: w536 -> [w553]
      tunnel: w535 -> [w556]
      tunnel: [w552] -> w530
      tunnel: [w551] -> w528
      tunnel: [w550] -> w529
      frame #0 {
        w537 = T6 6.5 items=["3 1/2"=3.5, "4 1/2"=4.5, "5 1/2"=5.5, "6 1/2"=6.5, "7 1/2"=7.5] ("Resolution in Digits")
        n269 = Fract/Exp String To Number(string="NI DMM 1 Voltage Range 4") -> (number=w542:dbl)  [unwired: 3 in, 1 out]
        n270 = call-poly <instrlib>:"niDMM Config Measurement.vi"("Range"=w542, "Resolution in Digits"=w537, "error in (no error)"=w543, "Function"=niDMM_Function."DC Volts" ("Measurement Type"), "instrument handle"=w539) -> ("error out"=w540:errorcluster, "instrument handle out"=w541:refnum<k15>)  [unwired: 5 in]
      }
      frame #1 {
        n271 = call <instrlib>:"niDMM Read.vi"("error in (no error)"=w556, "instrument handle"=w553) -> ("error out"=w550:errorcluster, "Measurement"=w545:dbl, "instrument handle out"=w551:refnum<k15>)  [unwired: 7 in]
        n272 = Fract/Exp String To Number(string="NI DMM 1 units 4") -> (number=w554:dbl)  [unwired: 3 in, 1 out]
        n273 = Multiply(x=w554, y=w545) -> (x*y=w547:dbl)
        n274 = Absolute Value(x=w547) -> (abs(x)=→"Voltage Char":dbl)
        n275 = Absolute Value(x=w547) -> (abs(x)=→"Voltage":dbl)
        n276 = Absolute Value(x=w545) -> (abs(x)=→"Voltage, V":dbl)
        n277 = local read "Стоп"() -> (w552:bool)
      }
    }
    n278 = call <vilib>:"Simple Error Handler.vi"("error in (no error)"=w529) -> ("error out"=w534:errorcluster)  [unwired: 1 in, 7 out]
  }
  n279 = invoke class="AmateurStepperMotor" method="Stop"(reference=w7) -> (reference out=w14:refnum<k24>, "Stop"=w15:refnum<k24>)  [unwired: 2 in, 1 out]
  n280 = property class="AmateurStepperMotor"(reference=w14, "HoldOn"=FALSE) -> (reference out=w13:refnum<k24>)  [unwired: 1 in, 1 out]
  n281 = invoke class="AmateurStepperMotor" method="Dispose"(reference=w13) -> (error out=w10:errorcluster)  [unwired: 2 in, 2 out]
  n282 = invoke class="SerialPort" method="Close"(reference=w20, error in=w10) -> (reference out=w9:refnum<k24>, error out=w11:errorcluster)  [unwired: 1 in, 1 out]
  n283 = invoke class="Task" method="Wait"(reference=w15) -> ()  [unwired: 2 in, 3 out]
  n284 = Close Reference(reference=w9, error in (no error)=w11) -> (error out=w12:errorcluster)
  n285 = call <vilib>:"Simple Error Handler.vi"("error in (no error)"=w12) -> ()  [unwired: 1 in, 8 out]
  n286 = VISA Close(VISA resource name=w18, error in (no error)=w17) -> (error out=w22:errorcluster)
  n287 = call <instrlib>:"niDMM Close.vi"("error in (no error)"=w29, "instrument handle"=w30) -> ()  [unwired: 9 in, 1 out]
  n288 = call <instrlib>:"niDCPower Close.vi"("instrument handle"=w34) -> ()  [unwired: 10 in, 1 out]
  n289 = call "Ophir Error Message.vi"("error in (no error)"=w22) -> ()  [unwired: 3 in, 4 out]
